vi "Video Processing.vi"() -> ()   [LabVIEW 2014]
uses:
  Global.vi
panel:
  in  "Prediction?":bool
  out "Image":T1(plugin-control)
  out "Video Loop":errorcluster
  out "Number of Particles before":i32
  out "Number of Particles after":i32
  in  "Number of Erosion":i32=30
  out "Video refresh":u32=48
  out "Read Video":errorcluster
  in  "milliseconds to wait":u32
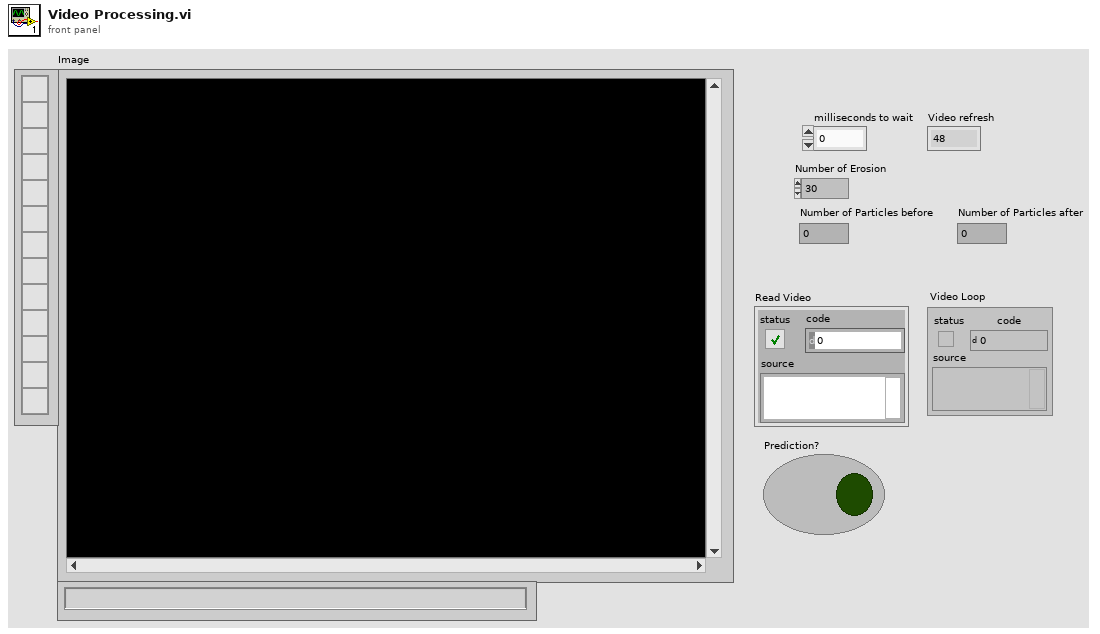
[diagram p1: front panel]
types:
  T1 = typedef "IMAQ Image.ctl" = refnum<image>
  T2 = cluster{"New Image":T1, "New Image":T1, "New Image":T1}
  T3 = cluster{"Left":dbl, "Top":dbl, "Right":dbl, "Bottom":dbl}
  T4 = cluster{"Horizontal position":dbl, "Verical position\n":dbl}
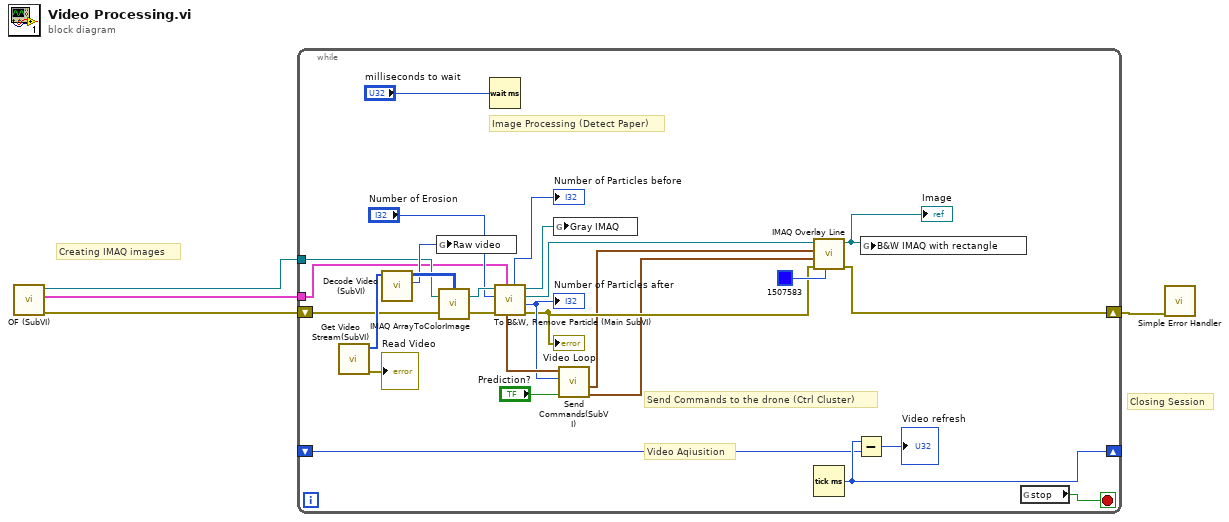
[diagram p0: block diagram]
diagram:
  # "Closing Session"
  # "Creating IMAQ images"
  n1 = call "OF (SubVI).vi"() -> ("error out"=w2:errorcluster, "Cluster"=w3:T2, "Refnum out"=w4:T1)  [unwired: 9 in]
  n2 = while {
    shift-right: [w27] -> _
    shift-left: _ -> [w26]
    tunnel: w4 -> [w15]
    tunnel: w3 -> [w14]
    shift-right: [w11] -> w1
    shift-left: w2 -> [w16]
    stop <- w17 stop-if-true
    # "Send Commands to the drone (Ctrl Cluster)"
    # "Image Processing (Detect Paper)"
    # "Video Aqiusition"
    n3 = call "Get Video Stream(SubVI).vi"() -> ("error out"=→"Read Video":errorcluster, "ImgData"=w30:u8[])  [unwired: 10 in]
    n4 = call "Decode Video (SubVI).vi"("ImgData"=w30) -> ("new picture"=w24:picture, "Array"=w28:u32[][])  [unwired: 9 in]
    n5 = global write "Global.vi" "Raw video"(w24) -> ()
    n6 = call "IMAQ ArrayToColorImage"("Image Pixels (U32)"=w28, "Image"=w15, "error in (no error)"=w16) -> ("Image Out"=w23:T1, "error out"=w22:errorcluster)  [unwired: 2 in]
    n7 = Wait (ms)(milliseconds to wait="milliseconds to wait") -> ()  [unwired: 1 out]
    n8 = call "To B&W, Remove Particle (Main SubVI).vi"("Image Reference Sources"=w14, "error in (no error)"=w22, "Number of Erosion"="Number of Erosion", "Refnum in"=w23) -> ("error out"=w10:errorcluster, "Number of Particles after"=w18:i32, "Image Out"=w7:T1, "Current Grayscale"=w13:T1, "Number of Particles before"=→"Number of Particles before":i32, "Cluster"=w20:T3)  [unwired: 1 in, 1 out]
    "Number of Particles after" <- w18
    "Video Loop" <- w10
    n9 = global write "Global.vi" "Gray IMAQ"(w13) -> ()
    n10 = call "Send Commands(SubVI).vi"("Prediction?"="Prediction?", "Number of Particles after"=w18, "Cluster"=w20) -> ("Predicted Position"=w8:T4, "Current position"=w9:T4)  [unwired: 7 in]
    n11 = call "IMAQ Overlay Line"("Color"=u32 1507583, "error in (no error)"=w10, "End Point"=w8, "Start Point"=w9, "Image"=w7) -> ("error out"=w11:errorcluster, "Image Out"=w5:T1)  [unwired: 5 in]
    "Image" <- w5
    n12 = Tick Count (ms)() -> (millisecond timer value=w27:u32)
    n13 = Subtract(x=w27, y=w26) -> (x-y=→"Video refresh":u32)
    n14 = global write "Global.vi" "B&W IMAQ with rectangle"(w5) -> ()
    n15 = global read "Global.vi" "stop"() -> (w17:bool)
  }
  n16 = call <vilib>:"Simple Error Handler.vi"("error in (no error)"=w1) -> ()  [unwired: 4 in, 5 out]
